vi "TopVI Ref FGV.vi"(7 "Action":enum16{"Read", "Write", "Other Action"}(ring), 8 "error in":errorcluster caption="error out", 11 "TopVI Ref":refnum<vi>) -> (0 "error out":errorcluster, 3 "TopVI Ref out":refnum<vi>)   [LabVIEW 2016]
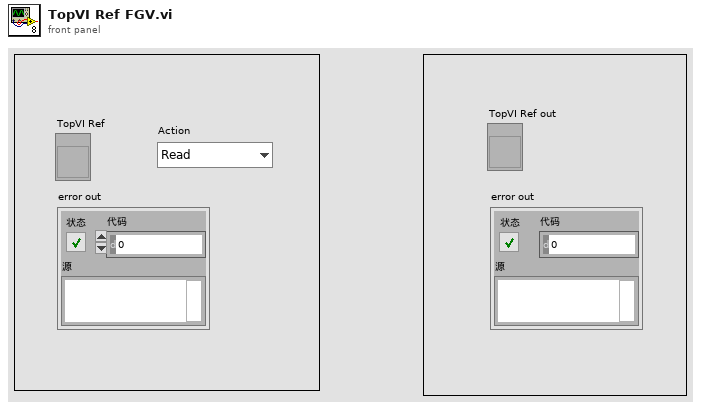
[diagram p1: front panel]
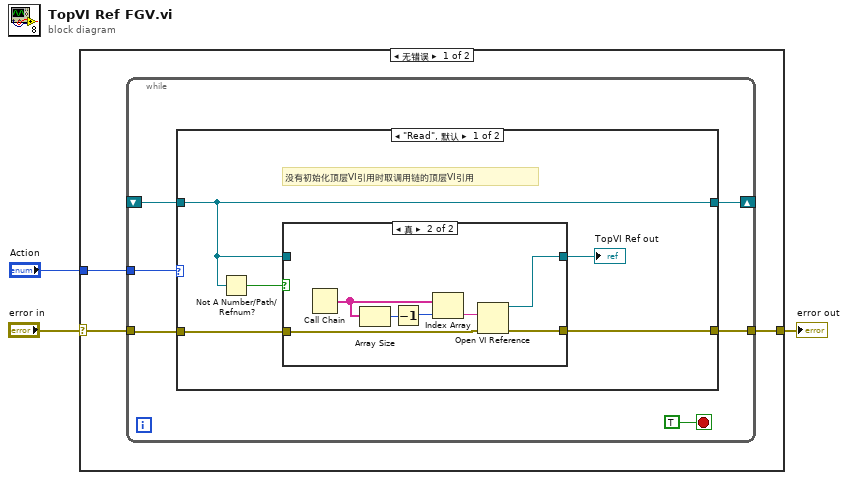
[diagram p0: block diagram]
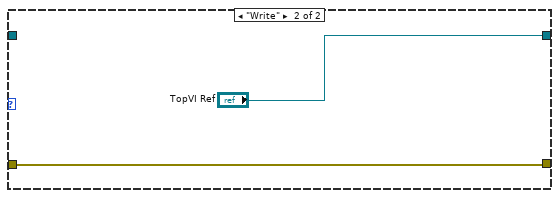
[diagram p3: hidden frame]
diagram:
  n1 = case shown="无错误" "error in" {
    selector: "error in" -> [w4 w29]
    tunnel: "Action" -> [w6 _]
    tunnel: [w5 w29] -> w2
    frame No Error {
      n2 = while {
        tunnel: w6 -> [w11]
        shift-right: [w10] -> _
        shift-left: _ -> [w9]
        tunnel: [w8] -> w5
        tunnel: w4 -> [w7]
        stop <- TRUE stop-if-true
        n3 = case shown="\"Read\", 默认" w11 {
          tunnel: [w16 "TopVI Ref"] -> w10
          tunnel: w9 -> [w16 _]
          tunnel: [w15 w27] -> w8
          tunnel: w7 -> [w14 w27]
          frame "Read", Default {
            # "没有初始化顶层VI引用时取调用链的顶层VI引用"
            n4 = Not A Number/Path/Refnum?(number/path/refnum=w16) -> (NaN/Path/Refnum?=w17:bool)
            n5 = case shown="真" w17 {
              tunnel: [w19 w22] -> w13
              tunnel: w16 -> [w19 _]
              tunnel: [w18 w21] -> w15
              tunnel: w14 -> [w18 w20]
              frame False {
              }
              frame True {
                n6 = Call Chain() -> (call chain=w26:string[])
                n7 = Array Size(array=w26) -> (size(s)=w25:i32)
                n8 = Decrement(x=w25) -> (x-1=w24:i32)
                n9 = Index Array(array=w26, index=w24) -> (element=w23:string)
                n10 = Open VI Reference(vi path=w23, error in (no error)=w20) -> (vi reference=w22:refnum<vi>, error out=w21:errorcluster)  [unwired: 4 in]
              }
            }
            "TopVI Ref out" <- w13
          }
          frame "Write" {
          }
        }
      }
    }
    frame Error {
    }
  }
  "error out" <- w2
